vi "GetErrorNum_8742.vi"(0 "CmdLib In":refnum<k24>, 5 "DeviceKey In":string, 7 "Device Address In":i32, 11 "error in (no error)":errorcluster) -> (4 "CmdLib Out":refnum<k24>, 6 "DeviceKey Out":string, 8 "Device Address Out":i32, 10 "Error Number":string, 15 "error out":errorcluster)   [LabVIEW 2009]
uses:
  C:/Code/Apps/Utilities/Picomotor/PicomotorApp/Install/Samples/LabVIEW/Mixed Devices/LabVIEW 2009/CmdLib8742.dll
panel:
  in  "number":string
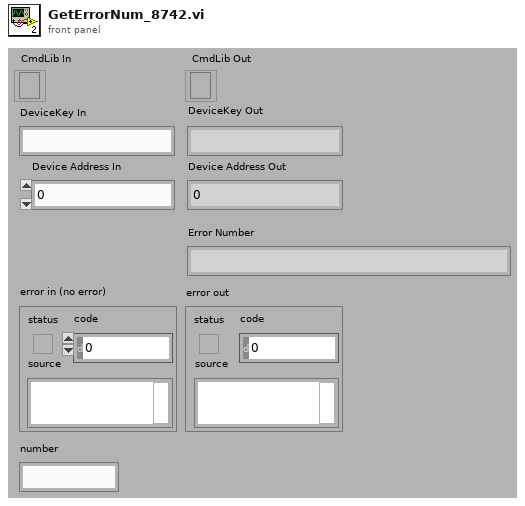
[diagram p1: front panel]
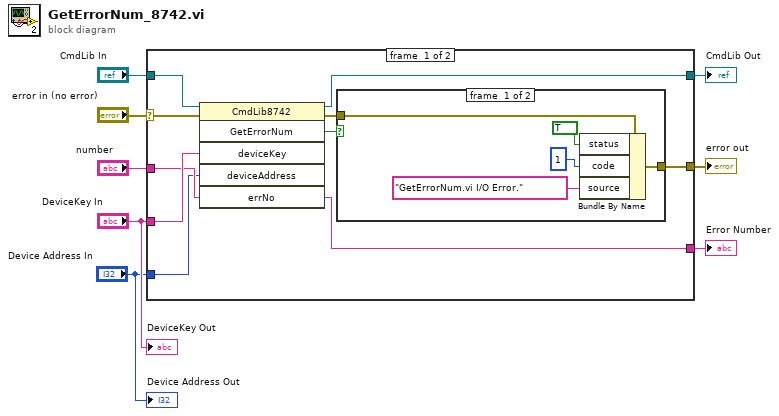
[diagram p0: block diagram]
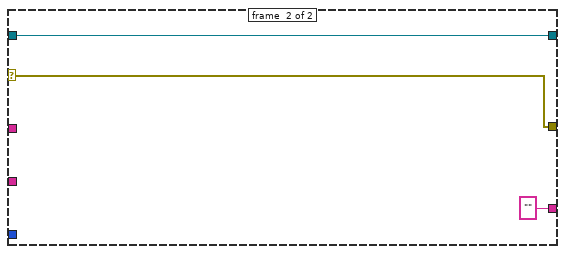
[diagram p3: hidden frame]
diagram:
  n1 = case shown="No Error" "error in (no error)" {
    selector: "error in (no error)" -> [w15 w25]
    tunnel: "CmdLib In" -> [w18 w27]
    tunnel: [w17 w27] -> w7
    tunnel: "number" -> [w11 _]
    tunnel: [w9 "" ("identification")] -> w5
    tunnel: "DeviceKey In" -> [w16 _]
    tunnel: [w12 w25] -> w2
    tunnel: "Device Address In" -> [w10 _]
    frame #0 {
      n2 = invoke class="CmdLib8742" method="GetErrorNum"(reference=w18, error in=w15, "deviceKey"=w16, "deviceAddress"=w10, "errNo"=w11) -> (reference out=w17:refnum<k24>, error out=w13:errorcluster, "GetErrorNum"=w14:bool, "errNo"=w9:string)  [unwired: 1 in, 2 out]
      n3 = case shown="False" w14 {
        tunnel: w13 -> [w23 w24]
        tunnel: [w22 w24] -> w12
        frame #0 {
          n4 = Bundle By Name(cluster=w23, "status"=TRUE, "code"=1, "source"="GetErrorNum.vi I/O Error.") -> (w22:errorcluster)
        }
        frame #1 {
        }
      }
    }
    frame #1 {
    }
  }
  "error out" <- w2
  "CmdLib Out" <- w7
  "Error Number" <- w5
  "DeviceKey Out" <- "DeviceKey In"
  "Device Address Out" <- "Device Address In"
